vi "TCPcloseConnection.vi"(0 "DashboardServer in":refnum<class "Dashboard Server.lvclass">, 5 "error in (no error)":errorcluster) -> (14 "DashboardServer out":refnum<class "Dashboard Server.lvclass">, 19 "error out":errorcluster)   [LabVIEW 2016, in "Dashboard Server.lvclass"]
uses:
  Dashboard Server.lvclass
  Dashboard Server.lvclass/Dashboard Server.ctl
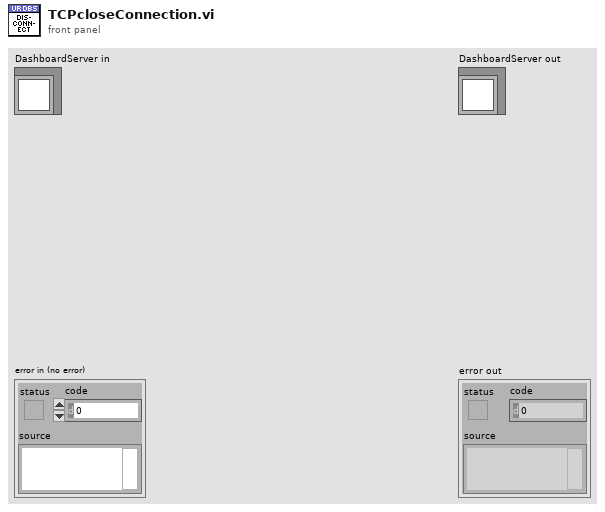
[diagram p1: front panel]
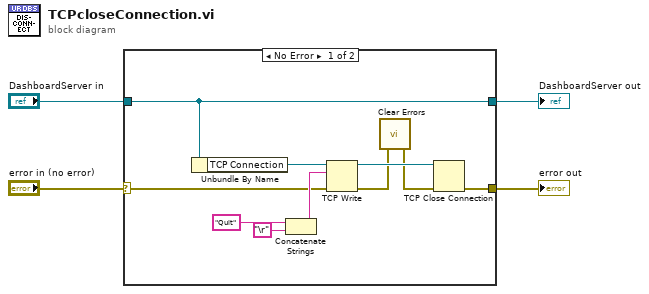
[diagram p0: block diagram]
diagram:
  n1 = case shown="No Error" "error in (no error)" {
    selector: "error in (no error)" -> [w8 w16]
    tunnel: [w14 w16] -> w3
    tunnel: [w13 w15] -> w1
    tunnel: "DashboardServer in" -> [w13 w15]
    frame No Error {
      n2 = Unbundle By Name(w13) -> ("TCP Connection"=w9:refnum<k5>)
      n3 = Concatenate Strings("Quit" ("string"), "\r") -> (w11:string)
      n4 = TCP Write(connection ID=w9, data in=w11, error in (no error)=w8) -> (connection ID out=w10:refnum<k5>, error out=w6:errorcluster)  [unwired: 1 in, 1 out]
      n5 = call <vilib>:"Clear Errors.vi"("error in (no error)"=w6) -> ("error out"=w5:errorcluster)  [unwired: 5 in, 1 out]
      n6 = TCP Close Connection(connection ID=w10, error in (no error)=w5) -> (error out=w14:errorcluster)  [unwired: 1 in, 1 out]
    }
    frame Error {
    }
  }
  "error out" <- w3
  "DashboardServer out" <- w1
